vi "PathPlanner_GridPosition_New.vi"(9 "Int Y":i32, 11 "Int X":i32) -> (3 "GridPosition":T1)   [LabVIEW 2019, in "PathPlanner24.lvlib"]
uses:
  PathPlanner24.lvlib
  TypeDef/PathPlannerFinderGridPosition.ctl
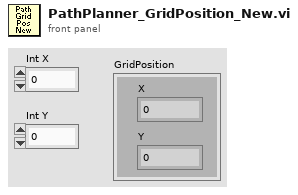
[diagram p1: front panel]
types:
  T1 = typedef "PathPlanner24.lvlib/PathPlannerFinderGridPosition.ctl" = cluster{"X":i32, "Y":i32}
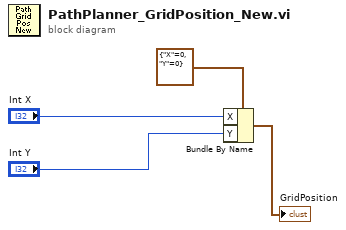
[diagram p0: block diagram]
diagram:
  n1 = Bundle By Name(cluster=T1 {"X"=0, "Y"=0} ("PathPlannerFinderGridPosition"), "X"="Int X", "Y"="Int Y") -> (→"GridPosition":T1)
